vi "readFromXML.vi"(8 "error in (no error)":errorcluster, 10 "XMLin":string, 11 "GuideAutoclearState in":refnum<class "GuideAutoclearState.lvclass">) -> (0 "error out":errorcluster, 3 "GuideAutoclearState out":refnum<class "GuideAutoclearState.lvclass">)   [LabVIEW 2022 SP3, in "TCSDataDefinitions.lvlib" / "TCSCommand.lvlib" / "GuiderCommands.lvlib" / "GuideAutoclearState.lvclass"]
uses:
  GuideAutoclearState.lvclass
  Enumerations/GuideAutoclearStateTypes.ctl
  GuideAutoclearState.lvclass/GuideAutoclearState.ctl
  GuiderCommands.lvclass
  <userlib>/Common/XML/XMLParser/XMLParser.lvclass
  TCSCommand.lvlib
panel:
  out "guideAutoClearStates":T1
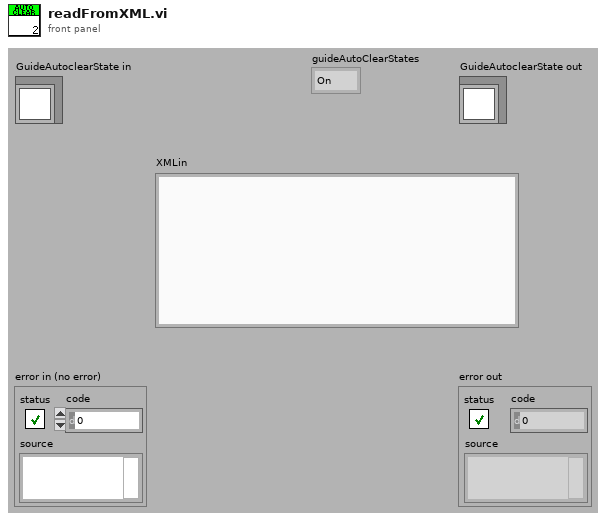
[diagram p1: front panel]
types:
  T1 = typedef "TCSDataDefinitions.lvlib/TCSCommand.lvlib/GuideAutoclearStateTypes.ctl" = enum16{"On", "Off"}
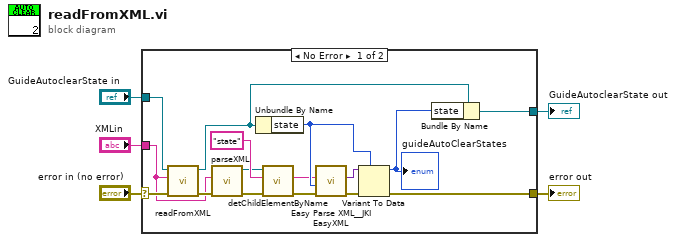
[diagram p0: block diagram]
diagram:
  n1 = case shown="No Error" "error in (no error)" {
    selector: "error in (no error)" -> [w17 w23]
    tunnel: [w16 w23] -> w4
    tunnel: [w14 w22] -> w2
    tunnel: "GuideAutoclearState in" -> [w21 w22]
    tunnel: "XMLin" -> [w10 _]
    frame No Error {
      n2 = call-parent "readFromXML.vi"("error in (no error)"=w17, "XMLin"=w10, "GuiderCommands in"=w21) -> ("error out"=w11:errorcluster, "GuiderCommands out"=w15:refnum<class "GuideAutoclearState.lvclass">)  [unwired: 7 in]
      n3 = call <userlib>:"parseXML.vi"("error in (no error)"=w11, "XMLString in"=w10) -> ("error out"=w12:errorcluster, "Element out"=w6:refnum<class "XMLParser.lvclass">)  [unwired: 8 in]
      n4 = Unbundle By Name(w15) -> ("state"=w20:T1)
      n5 = call <userlib>:"detChildElementByName.vi"("error in (no error)"=w12, "childName"="state" ("ChildName"), "Element in"=w6) -> ("error out"=w7:errorcluster, "childXML"=w8:string)  [unwired: 5 in, 2 out]
      n6 = call <vilib>:"Easy Parse XML__JKI EasyXML.vi"("error in (no error)"=w7, "LabVIEW Data (Type)"=w20, "XML String"=w8) -> ("error out"=w18:errorcluster, "LabVIEW Data"=w19:variant)  [unwired: 7 in]
      n7 = Variant To Data(error in=w18, type=w20, Variant=w19) -> (data=w13:T1, error out=w16:errorcluster)
      "guideAutoClearStates" <- w13
      n8 = Bundle By Name(cluster=w15, "state"=w13) -> (w14:refnum<class "GuideAutoclearState.lvclass">)
    }
    frame Error {
    }
  }
  "error out" <- w4
  "GuideAutoclearState out" <- w2
